vi "Check.vi"(8 "error in (no error)":errorcluster, 11 "Pointer in":refnum<class "Pointer.lvclass">) -> (0 "error out":errorcluster, 2 "LabVIEW pointer?":bool, 3 "Pointer out":refnum<class "Pointer.lvclass">)   [LabVIEW 2020, in "Memory Manager.lvlib" / "Pointer.lvclass"]
doc: "Checks that the provided <b>pointer</b> was allocated by LabVIEW."
uses:
  Pointer.lvclass
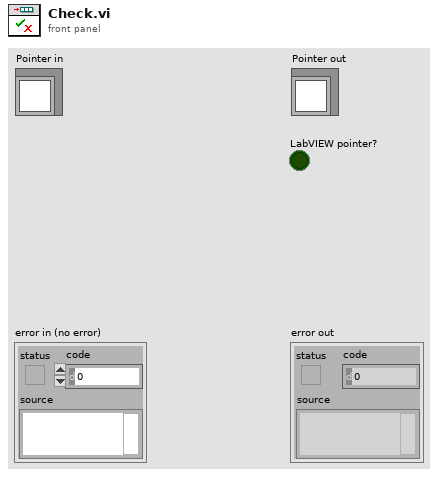
[diagram p1: front panel]
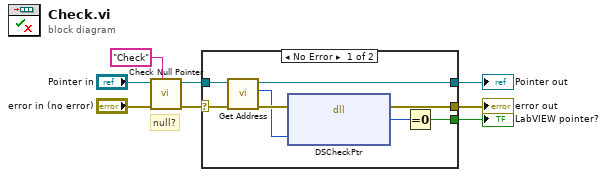
[diagram p0: block diagram]
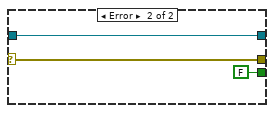
[diagram p2: hidden frame]
diagram:
  # "null?"
  n1 = call "Check Null Pointer.vi"("source vi name"="Check", "error in (no error)"="error in (no error)", "Pointer in"="Pointer in") -> ("error out"=w1:errorcluster, "Pointer out"=w3:refnum<class "Pointer.lvclass">)  [unwired: 7 in]
  n2 = case shown="No Error" w1 {
    selector: w1 -> [w10 w17]
    tunnel: [w15 w18] -> w8
    tunnel: [w14 w17] -> w7
    tunnel: [w12 FALSE] -> w6
    tunnel: w3 -> [w11 w18]
    frame No Error {
      n3 = call "Get Address.vi"("Pointer in"=w11) -> ("address"=w9:u64, "Pointer out"=w15:refnum<class "Pointer.lvclass">)  [unwired: 9 in]
      n4 = dll-call lib="LabVIEW" fn="DSCheckPtr"(error in=w10, "pointer"=w9) -> (error out=w14:errorcluster, "return"=w13:i32)  [unwired: 3 in, 1 out]
      n5 = Equal To 0?(x=w13) -> (x = 0?=w12:bool)
    }
    frame Error {
    }
  }
  "error out" <- w7
  "Pointer out" <- w8
  "LabVIEW pointer?" <- w6
